vi "In-Range (ARGB).vi"(8 "error in (no error)":errorcluster, 9 "In-Range Image Colour Range":T1, 10 "In-Range-Result in":T2, 11 "ARGB Image Source in":T3) -> (0 "error out":errorcluster, 3 "In-Range-Result":T2)   [LabVIEW 2020, in "image.lvlib"]
doc: "Compute a single channel image which will contain non-zero pixels for any pixel in the Source Image which is between the two Pixel Values specified. The range values are interpolated using the HSV colour-space.\n\nThis is similar to Image \"Match-Value\" except it matches between an upper and lower value."
uses:
  image.lvlib
  ARGB Image.ctl
  Greyscale Image.ctl
  In-Range Image Colour Range.ctl
  ffccc43a-a069-4092-9152-56f2c6e40fec.vi
  <vilib>/Utility/error.llb/Error Cluster From Error Code.vi
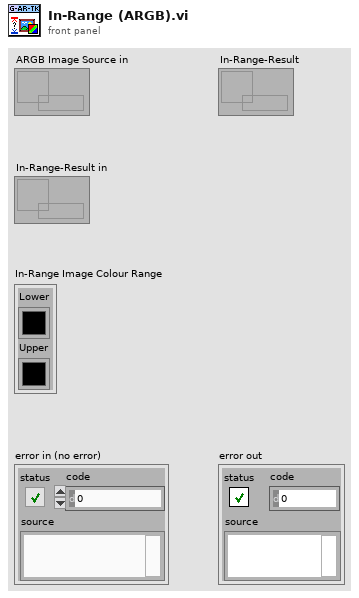
[diagram p1: front panel]
types:
  T1 = typedef "image.lvlib/In-Range Image Colour Range.ctl" = cluster{"Lower":u32, "Upper":u32}
  T2 = typedef "image.lvlib/Greyscale Image.ctl" = refnum<data-value>
  T3 = typedef "image.lvlib/ARGB Image.ctl" = refnum<data-value>
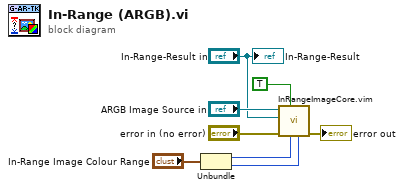
[diagram p0: block diagram]
diagram:
  n1 = Unbundle("In-Range Image Colour Range") -> ("Lower"=w6:u32, "Upper"=w5:u32)
  n2 = call "InRangeImageCore.vim"("Upper"=w5, "Lower"=w6, "IgnoreAlpha"=TRUE, "error in (no error)"="error in (no error)", "In-Range-Result"="In-Range-Result in", "Src"="ARGB Image Source in") -> ("error out"=→"error out":errorcluster)  [unwired: 5 in]
  "In-Range-Result" <- "In-Range-Result in"
